vi "Get Series Graph.vi"(11 "Series Graph in":refnum<class "Graph with Series View.lvclass">) -> (2 "Series Graph":refnum<vi>, 3 "Series Graph out":refnum<class "Graph with Series View.lvclass">)   [LabVIEW 2023, in "Graph with Series View.lvclass"]
uses:
  Graph with Series View.lvclass
  Graph with Series View.lvclass/Graph with Series View.ctl
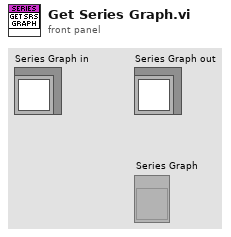
[diagram p1: front panel]
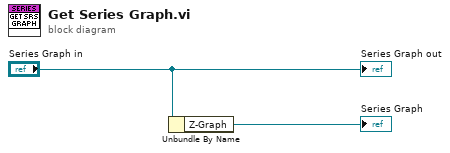
[diagram p0: block diagram]
diagram:
  n1 = Unbundle By Name("Series Graph in") -> ("Z-Graph"=→"Series Graph":refnum<vi>)
  "Series Graph out" <- "Series Graph in"
